vi "MES操作函数-Upload.vi"(5 "测试结果":string="产品名称：SA 左前玻璃升降器\n测试程序版本：150113-A0\n测试时间：\n,,!测试步骤,判定条件,测试值!上电,-,电压：14.0V 限流：1.0A!软件版本号,{06 50 01 00 32 01 F4 AA;\n03 7F 2F 31 AA AA AA AA},06 50 01 00 32 01 F4 AA \n03 7F 2F 31 AA AA AA AA ;!中控锁上锁,{01 AA 02 A4 86 01 01},00 AA 02 A4 86 01 01 90 ，不合格!", 7 "SN":string="0105442MF011400002", 8 "error in (no error)":errorcluster caption="错误输入（无错误）", 10 "总结果（测试）":bool, 11 "MES配置":T1={"接口地址："="http://10.9.30.175:50100/manufacturing/IntegrationServlet?InterType=XML&message=", "SITE（站点）   "="A157", "PWD（口令）"="123456", "RESOURCE（资源）"="A-6-Z-TEST", "OPERATION（工序）"="Z-TEST", "USER（用户）"="TEST", "QTY"="", "ACTIVITY"="", "NC_CODE（NG代码）"="", "启用MES"=TRUE}) -> (0 "error out":errorcluster caption="错误输出", 3 "Y":bool)   [LabVIEW 2011]
panel:
  out "数组":string[](array[string])
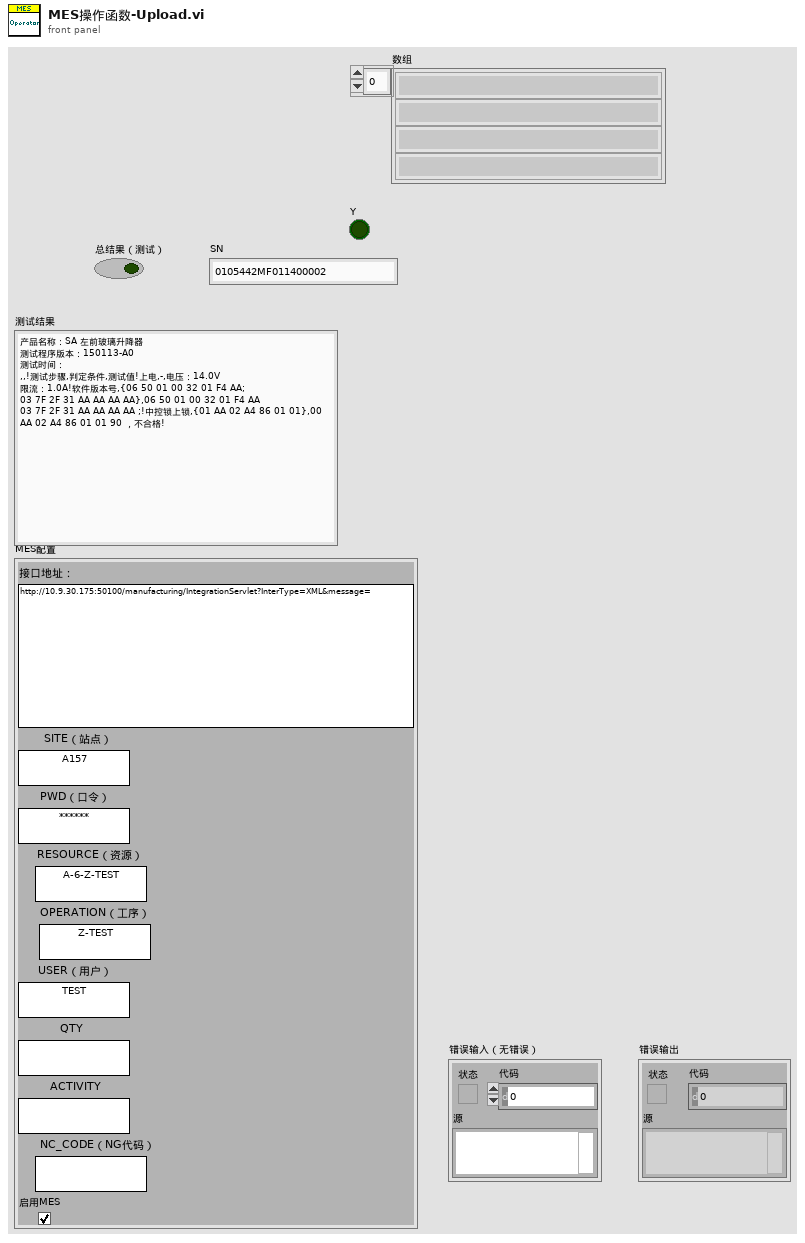
[diagram p1: front panel]
types:
  T1 = typedef "MES设置.ctl" = cluster{"接口地址：":string, "SITE（站点）   ":string, "PWD（口令）":string, "RESOURCE（资源）":string, "OPERATION（工序）":string, "USER（用户）":string, "QTY":string, "ACTIVITY":string, "NC_CODE（NG代码）":string, "启用MES":bool}
  T2 = enum16{"USER_CHECK", "SFC_CHECK", "RLT_PASS", "RLT_ERROR", "RES_AREA"}
  T3 = cluster{"接口地址：":string, "默认值 1":i32, "接口地址：":string}
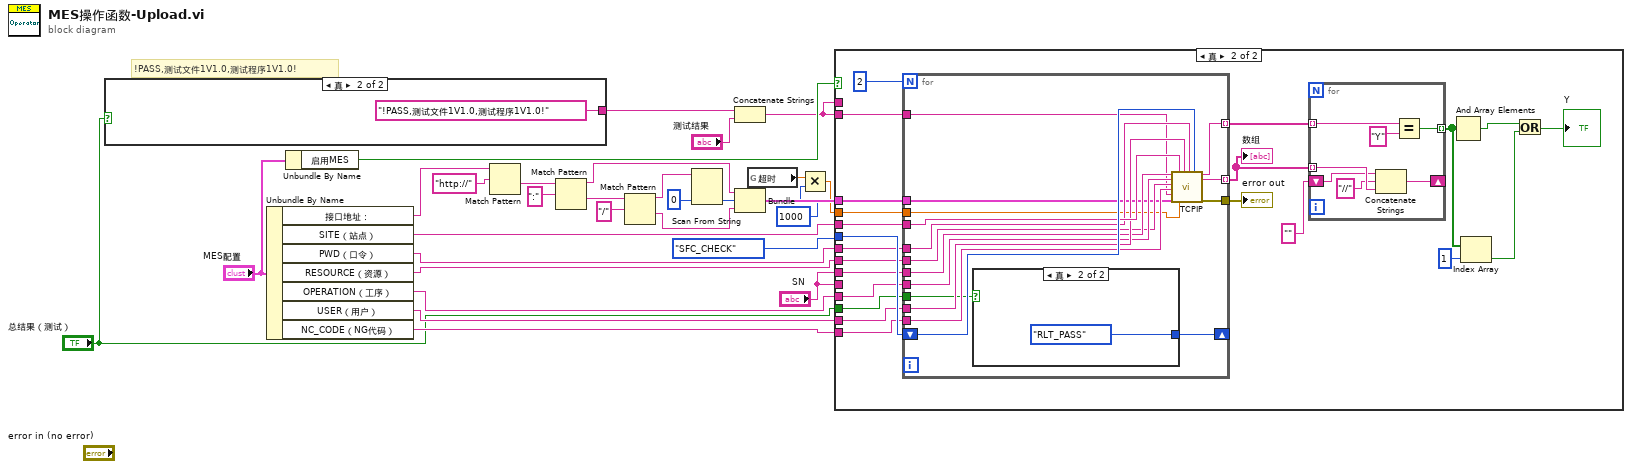
[diagram p0: block diagram]
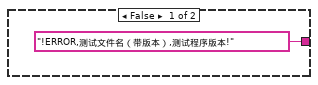
[diagram p2: hidden frame]
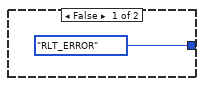
[diagram p4: hidden frame]
diagram:
  # "!PASS,测试文件1V1.0,测试程序1V1.0!"
  n1 = case shown="真" "总结果（测试）" {
    tunnel: ["!ERROR,测试文件名（带版本）,测试程序版本!" ("字符串") "!PASS,测试文件1V1.0,测试程序1V1.0!" ("字符串")] -> w6
    frame False {
    }
    frame True {
    }
  }
  n2 = Unbundle By Name("MES配置") -> ("接口地址："=w20:string, "SITE（站点）"=w27:string, "PWD（口令）"=w25:string, "RESOURCE（资源）"=w23:string, "OPERATION（工序）"=w24:string, "USER（用户）"=w26:string, "NC_CODE（NG代码）"=w22:string)
  n3 = Unbundle By Name("MES配置") -> ("启用MES"=w8:bool)
  n4 = Match Pattern(string=w20, regular expression="http://" ("正则表达式")) -> (after substring=w18:string)  [unwired: 1 in, 3 out]
  n5 = Match Pattern(string=w18, regular expression=":" ("正则表达式")) -> (before substring=w12:string, after substring=w16:string)  [unwired: 1 in, 2 out]
  n6 = Match Pattern(string=w16, regular expression="/" ("正则表达式")) -> (before substring=w13:string, after substring=w14:string)  [unwired: 1 in, 2 out]
  n7 = Scan From String(input string=w13, default 1=0 ("默认值 1")) -> (output 1=w10:i32)  [unwired: 3 in, 3 out]
  n8 = Concatenate Strings(w6, "测试结果") -> (w5:string)
  n9 = Bundle("接口地址："=w12, "默认值 1"=w10, "接口地址："=w14) -> (w11:T3)  [unwired: 1 in]
  n10 = global read "全局 TCPIP超时.vi" "超时"() -> (w3:dbl)
  n11 = Multiply(x=w3, y=u64 1000 ("TCP超时")) -> (x*y=w1:dbl)
  n12 = case shown="真" w8 {
    tunnel: T2."SFC_CHECK" ("STATE") -> [_ w53]
    tunnel: w27 -> [_ w52]
    tunnel: w26 -> [_ w51]
    tunnel: w25 -> [_ w50]
    tunnel: "SN" -> [_ w49]
    tunnel: w24 -> [_ w48]
    tunnel: w23 -> [_ w47]
    tunnel: w22 -> [_ w46]
    tunnel: w1 -> [_ w45]
    tunnel: w5 -> [_ w44]
    tunnel: w11 -> [_ w43]
    tunnel: "总结果（测试）" -> [_ w41]
    tunnel: w5 -> [_ _]
    tunnel: "SN" -> [_ _]
    frame False {
    }
    frame True {
      n13 = for {
        N: 2 -> [_]
        tunnel: w52 -> [w75]
        tunnel: w51 -> [w74]
        tunnel: w50 -> [w73]
        tunnel: w49 -> [w72]
        tunnel: w48 -> [w71]
        tunnel: w47 -> [w70]
        tunnel: w46 -> [w69]
        tunnel: w45 -> [w68]
        tunnel: w44 -> [w67]
        tunnel: w43 -> [w66]
        shift-right: [w64] -> _
        shift-left: w53 -> [w76]
        tunnel: w41 -> [w65]
        tunnel: [w63] -> w39 mode=indexing
        tunnel: [w62] -> w40 mode=indexing
        tunnel: [w61] -> w37
        n14 = case shown="真" w65 {
          tunnel: [T2."RLT_ERROR" ("STATE") T2."RLT_PASS" ("STATE")] -> w64
          frame False {
          }
          frame True {
          }
        }
        n15 = call "TCPIP.vi"("SFC"=w72, "OPERATOR"=w71, "RESOURCE"=w70, "NC_CODE"=w69, "TESTRLT"=w67, "SERVER"=w66, "SITE"=w75, "TCP超时"=w68, "USER"=w74, "PWD"=w73, "STATE"=w76) -> ("Y&N"=w62:string, "系统消息"=w63:string, "error out"=w61:errorcluster)  [unwired: 6 in]
      }
      "数组" <- w39
      "error out" <- w37
      n16 = for {
        tunnel: w40 -> [w60] mode=indexing
        tunnel: [w58] -> w36 mode=indexing
        tunnel: w39 -> [w57] mode=indexing
        shift-right: [w56] -> _
        shift-left: "" -> [w55]
        n17 = Concatenate Strings(w55, "//" ("字符串"), w57) -> (w56:string)
        n18 = Equal?(x=w60, y="Y") -> (x = y?=w58:bool)
      }
      n19 = And Array Elements(Boolean array=w36) -> (logical AND=w33:bool)
      n20 = Index Array(array=w36, index=1 ("索引")) -> (element=w32:bool)
      n21 = Or(x=w33, y=w32) -> (x .or. y?=→"Y":bool)
    }
  }
